vi "InRange (SubVI).vi"(6 "Threshold":dbl, 9 "Boat Position":T1, 10 "y":dbl, 11 "x":dbl) -> (3 "In Range?":bool)   [LabVIEW 2011]
uses:
  Position.ctl
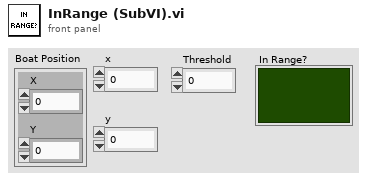
[diagram p1: front panel]
types:
  T1 = typedef "Position.ctl" = cluster{"X":sgl, "Y":sgl}
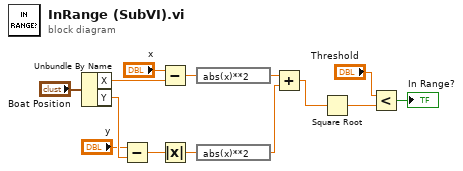
[diagram p0: block diagram]
diagram:
  n1 = Unbundle By Name("Boat Position") -> ("X"=w2:sgl, "Y"=w5:sgl)
  n2 = Subtract(x="y", y=w5) -> (x-y=w6:dbl)
  n3 = Subtract(x="x", y=w2) -> (x-y=w7:dbl)
  n4 = Absolute Value(x=w6) -> (abs(x)=w8:dbl)
  n5 = expression code="abs(x)**2"(w7) -> (w9:dbl)
  n6 = expression code="abs(x)**2"(w8) -> (w10:dbl)
  n7 = Add(x=w9, y=w10) -> (x+y=w11:dbl)
  n8 = Square Root(x=w11) -> (sqrt(x)=w12:dbl)
  n9 = Less?(x="Threshold", y=w12) -> (x < y?=→"In Range?":bool)
